vi "tm_initialize.vi"(8 "error in (no error)":errorcluster {"code" format="%.0x"}) -> (0 "error out":errorcluster {"code" format="%.0x"}, 1 "Camera Details Array":T2(array[cluster]), 2 "Version Info":T1, 3 "Number Of Cameras":u32)   [LabVIEW 2015]
uses:
  tmcamcon.dll
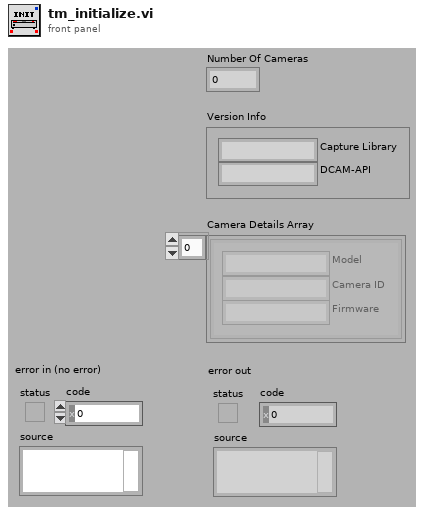
[diagram p1: front panel]
types:
  T1 = cluster{"Capture Library":string, "DCAM-API":string}
  T2 = cluster{"Model":string, "Camera ID":string, "Firmware":string}[]
  T3 = cluster{"string":string, "string":string, "string":string}
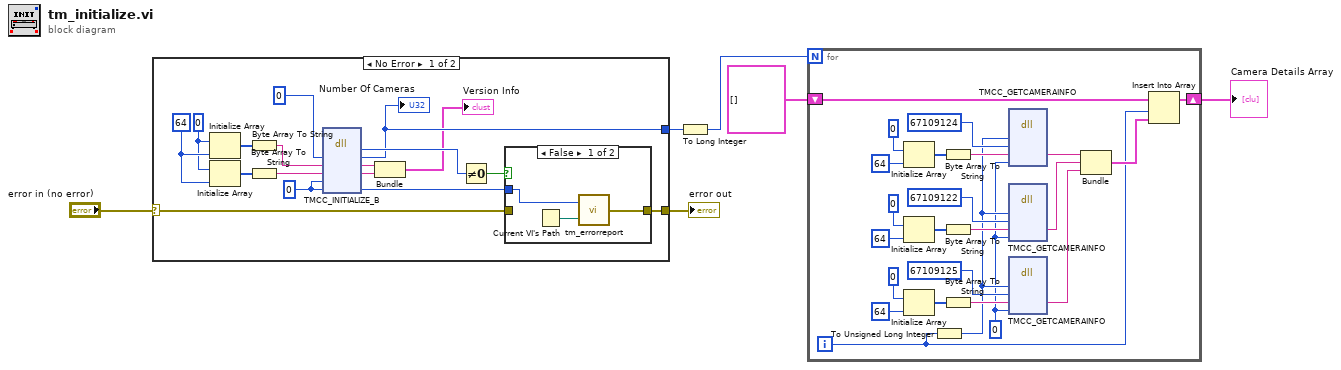
[diagram p0: block diagram]
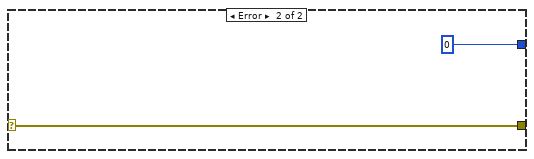
[diagram p3: hidden frame]
diagram:
  n1 = case shown="No Error" "error in (no error)" {
    selector: "error in (no error)" -> [w22 w29]
    tunnel: [w21 w29] -> w3
    tunnel: [w17 u32 0] -> w5
    frame No Error {
      w11 = 64
      w10 = u8 0
      w14 = 0 ("Erval")
      n2 = Initialize Array(w10, w11) -> (w16:u8[])
      n3 = Initialize Array(w10, w11) -> (w15:u8[])
      n4 = Byte Array To String(unsigned byte array=w16) -> (string=w12:string)
      n5 = Byte Array To String(unsigned byte array=w15) -> (string=w13:string)
      n6 = dll-call lib="tmcamcon.dll" fn="TMCC_INITIALIZE_B"("Count"=u32 0, "tmver"=w12, "dcamver"=w13, "Force"=w14, "Erval"=w14) -> ("return type"=w18:u32, "Count"=w17:u32, "tmver"=w9:string, "dcamver"=w8:string, "Erval"=w23:i32)  [unwired: 4 in, 2 out]
      "Number Of Cameras" <- w17
      n7 = Bundle("tmver"=w9, "dcamver"=w8) -> (→"Version Info":cluster{"tmver":string, "dcamver":string})  [unwired: 1 in]
      n8 = Not Equal To 0?(x=w18) -> (x != 0?=w19:bool)
      n9 = case shown="False" w19 {
        tunnel: w22 -> [_ w27]
        tunnel: [w26 w27] -> w21
        tunnel: w23 -> [w24 _]
        frame False {
          n10 = Current VI's Path() -> (path=w25:path)
          n11 = call "tm_errorreport.vi"("Source"=w25, "Error"=w24) -> ("error out"=w26:errorcluster)
        }
        frame True {
        }
      }
    }
    frame Error {
    }
  }
  "error out" <- w3
  n12 = To Long Integer(number=w5) -> (32bit integer=w4:i32)
  n13 = for {
    N: w4 -> [_]
    shift-right: [w34] -> w1
    shift-left: T2 [] ("Camera Details Array") -> [w35]
    i -> [w32]
    w30 = 0 ("Erval")
    n14 = Initialize Array(u8 0, 64) -> (w53:u8[])
    n15 = Initialize Array(u8 0, 64) -> (w48:u8[])
    n16 = Initialize Array(u8 0, 64) -> (w43:u8[])
    n17 = To Unsigned Long Integer(number=w32) -> (unsigned 32bit integer=w31:u32)
    n18 = Byte Array To String(unsigned byte array=w53) -> (string=w49:string)
    n19 = Byte Array To String(unsigned byte array=w48) -> (string=w44:string)
    n20 = Byte Array To String(unsigned byte array=w43) -> (string=w39:string)
    n21 = dll-call lib="tmcamcon.dll" fn="TMCC_GETCAMERAINFO"("index"=w31, "ID"=u32 67109124, "string"=w49, "Erval"=w30) -> ("string"=w38:string)  [unwired: 7 in, 2 out]
    n22 = dll-call lib="tmcamcon.dll" fn="TMCC_GETCAMERAINFO"("index"=w31, "ID"=u32 67109122, "string"=w44, "Erval"=w30) -> ("string"=w37:string)  [unwired: 7 in, 2 out]
    n23 = dll-call lib="tmcamcon.dll" fn="TMCC_GETCAMERAINFO"("index"=w31, "ID"=u32 67109125, "string"=w39, "Erval"=w30) -> ("string"=w36:string)  [unwired: 7 in, 2 out]
    n24 = Bundle("string"=w38, "string"=w37, "string"=w36) -> (w33:T3)  [unwired: 1 in]
    n25 = Insert Into Array(array=w35, index=w32, new element=w33) -> (w34:T2)
  }
  "Camera Details Array" <- w1
